vi "SPI read words.vi"(7 "Number of words":i32=3, 8 "error in (no error)":errorcluster, 9 "address":u8, 10 "spi configuration in":T2, 11 "Refnum in":T1) -> (0 "error out":errorcluster, 1 "data out":i16[](array[numeric]), 2 "spi configuration out":T2, 3 "Refnum out":T1)   [LabVIEW 2013]
uses:
  <vilib>/ni845x/ni845x.llb/ni845xSpiConfiguration.ctl
  <vilib>/ni845x/ni845x.llb/ni845xControl.ctl
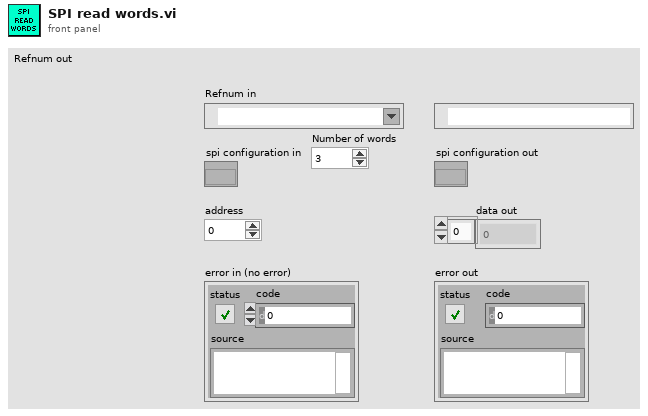
[diagram p1: front panel]
types:
  T1 = typedef "ni845xControl.ctl" = refnum<k21>
  T2 = typedef "ni845xSpiConfiguration.ctl" = refnum<k20>
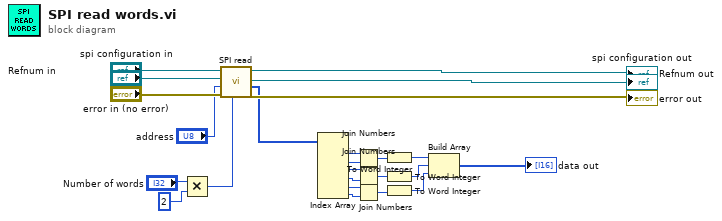
[diagram p0: block diagram]
diagram:
  n1 = Multiply(x="Number of words", y=2 ("x")) -> (x*y=w2:i32)
  n2 = call "SPI read.vi"("Number of bytes"=w2, "error in (no error)"="error in (no error)", "Address"="address", "spi configuration in"="spi configuration in", "Device ref in"="Refnum in") -> ("error out"=→"error out":errorcluster, "read data"=w15:u8[], "spi configuration out"=→"spi configuration out":T2, "Device ref out"=→"Refnum out":T1)  [unwired: 3 in]
  n3 = Index Array(array=w15) -> (element #1=w4:u8, element #2=w3:u8, element #3=w7:u8, element #4=w5:u8, element #5=w8:u8, element #6=w6:u8)  [unwired: 6 in]
  n4 = Join Numbers(hi=w4, lo=w3) -> ((hi.lo)=w9:u16)
  n5 = Join Numbers(hi=w7, lo=w5) -> ((hi.lo)=w10:u16)
  n6 = Join Numbers(hi=w8, lo=w6) -> ((hi.lo)=w11:u16)
  n7 = To Word Integer(number=w9) -> (16bit integer=w12:i16)
  n8 = To Word Integer(number=w10) -> (16bit integer=w13:i16)
  n9 = To Word Integer(number=w11) -> (16bit integer=w14:i16)
  n10 = Build Array(w12, w13, w14) -> (→"data out":i16[])
